vi "Choreo_ChoreoDifferential_LoadAllTrajectories.vi"(8 "error in (no error)":errorcluster) -> (0 "error out":errorcluster, 3 "Trajectories":string[](array[string]))   [LabVIEW 2019, in "ChoreoLib.lvlib"]
doc: "Load all *.traj files found in the default choreo deploy directory into cache. This is an easy way to load everything into memory when the robot is started. All trajectories are expected to be of type Differential.\n\n\nInputs:\n - ErrorIn - cluster - standard error cluster. Can be used to force execution order.\n\nOutputs:\n - Trajectories - string array - List of the names of the trajectories found and loaded. This is just for information.\n - ErrorOut - cluster - standard error cluster. Can be used to force execution order and check for errors."
uses:
  ChoreoLib.lvlib
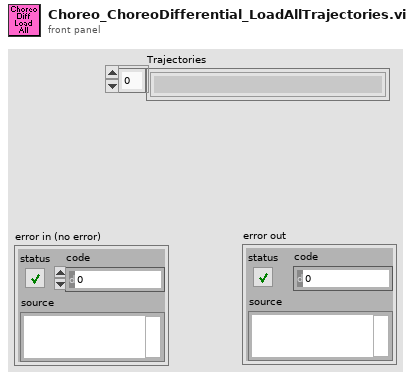
[diagram p1: front panel]
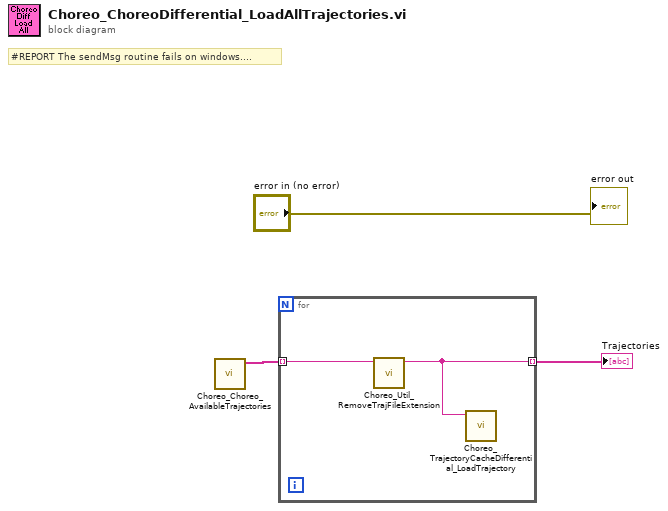
[diagram p0: block diagram]
diagram:
  # "#REPORT The sendMsg routine fails on windows...."
  n1 = call "Choreo_Choreo_AvailableTrajectories.vi"() -> ("filenames"=w3:string[])  [unwired: 9 in, 2 out]
  n2 = for {
    tunnel: w3 -> [w4] mode=indexing
    tunnel: [w5] -> w2 mode=indexing
    n3 = call "Choreo_Util_RemoveTrajFileExtension.vi"("FileNameIn"=w4) -> ("FileNameOut"=w5:string)  [unwired: 10 in]
    n4 = call "Choreo_TrajectoryCacheDifferential_LoadTrajectory.vi"("TrajectoryName"=w5) -> ()  [unwired: 9 in, 2 out]
  }
  "Trajectories" <- w2
  "error out" <- "error in (no error)"
